vi "fpga_ARC Core (32ch).vi"(0 "data input":i32, 1 "ARC Constants":T3={"bufsize"=512, "bufsize-1"=511, "NChan"=8, "NChan-1"=7, "1/2SymPeriods"=10, "Neg1/2SymPeriods"=-10, "polyOrder-1"=4, "maxDec-1"=24}, 2 "timestamp&count":T1 {"TAI timestamp" format="%.42g"}, 5 "data valid":bool, 7 "resample position [U64.16]":fxp<+,64,16>, 9 "stepsize [U64.8]":fxp<+,64,8>, 11 "position valid":bool, 12 "Ready for output":bool, 13 "Frequency":fxp<+,32,8> format="%.27g") -> (3 "FIFO timeout?":bool, 4 "resample data":T2 {"frequency" format="%.59g"; "Resample position" format="%.53g"; "even-angle signal" format="%.30g"}, 6 "timestamp&count":T1, 8 "muti_ch position valid?":bool, 14 "ready for input":bool, 15 "output valid":bool)   [LabVIEW 2014, in "NI_EP_Resample_FPGA.lvlib"]
uses:
  <vilib>/addons/Electrical Power/PQ/Resampling/NI_EP_Resample_FPGA.lvlib
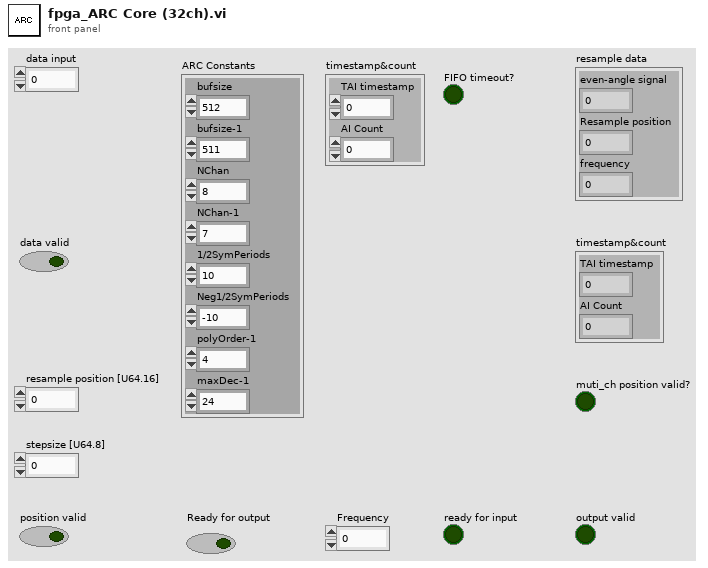
[diagram p1: front panel]
types:
  T1 = cluster{"TAI timestamp":fxp<+,64,32>, "AI Count":u16}
  T2 = cluster{"even-angle signal":fxp<+/-,32,3>, "Resample position":fxp<+,64,16>, "frequency":fxp<+,32,8>}
  T3 = cluster{"bufsize":u16, "bufsize-1":u16, "NChan":u8, "NChan-1":u8, "1/2SymPeriods":i8, "Neg1/2SymPeriods":i8, "polyOrder-1":u8, "maxDec-1":u8}
  T4 = cluster{"sample position":u16, "coef [I32.2]":fxp<+/-,32,2>, "last tap":bool}
  T5 = cluster{"even-angle signal[I32.3]":fxp<+/-,32,3>, "resample position":fxp<+,64,16>, "frequency":fxp<+,32,8>}
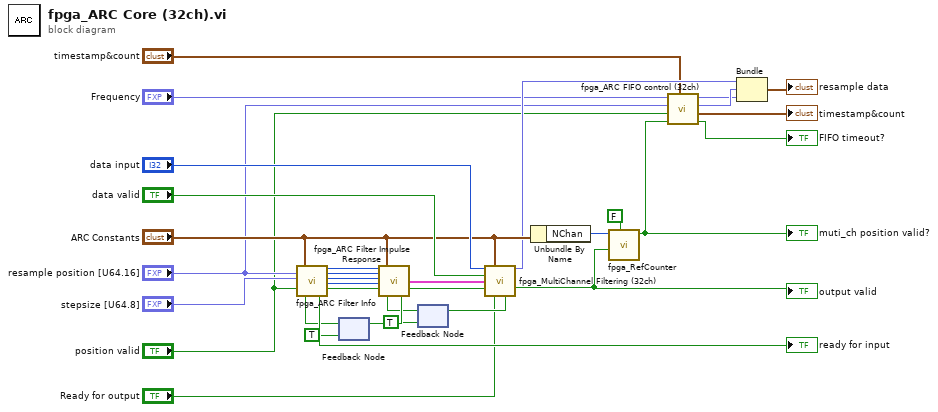
[diagram p0: block diagram]
diagram:
  n1 = feedback #1(TRUE ("ready for input")) -> (w30:bool)
  n2 = call <vilib>:"fpga_ARC Filter Info.vi"("resample position [U64.16]"="resample position [U64.16]", "stepsize [U64.8]"="stepsize [U64.8]", "input valid"="position valid", "ARC Constants"="ARC Constants", "ready for output"=w30) -> ("ready for input"=→"ready for input":bool, "Initial position"=w28:u16, "Initial offset"=w32:u32, "Number of taps"=w26:u16, "filterStepSize[U32.0]"=w31:u32, "output valid"=w27:bool)  [unwired: 1 in, 8 out]
  n3 = feedback #2(TRUE ("ready for filter")) -> (w25:bool)
  n4 = call <vilib>:"fpga_ARC Filter Impulse Response.vi"("Initial position"=w28, "Initial offset"=w32, "Number of taps"=w26, "filterStepSize[U32.0]"=w31, "input valid"=w27, "ARC Constants"="ARC Constants", "ready for output"=w25) -> ("ready for input"=w29:bool, "filter info"=w22:T4, "output valid"=w23:bool)  [unwired: 10 out]
  n5 = feedback-in #1(w29) -> ()
  n6 = call <vilib>:"fpga_MultiChannel Filtering (32ch).vi"("data input"="data input", "ARC Constants"="ARC Constants", "data valid"="data valid", "filter info"=w22, "filter valid"=w23, "Ready for output"="Ready for output") -> ("even-angle signal[I32.3]"=w13:fxp<+/-,32,3>, "output valid"=w10:bool, "ready for filter"=w24:bool)  [unwired: 7 in]
  "output valid" <- w10
  n7 = feedback-in #2(w24) -> ()
  n8 = Unbundle By Name("ARC Constants") -> ("NChan"=w12:u8)
  n9 = call <vilib>:"fpga_RefCounter.vi"("reset"=FALSE, "input valid?"=w10, "NChan"=w12) -> ("Multichannel enable"=w6:bool)  [unwired: 7 in, 1 out]
  "muti_ch position valid?" <- w6
  n10 = call <vilib>:"fpga_ARC FIFO control (32ch).vi"("timestamp&count"="timestamp&count", "Read FIFO"=w6, "write FIFO"="position valid", "resample position"="resample position [U64.16]", "frequency"="Frequency") -> ("FIFO time out?"=→"FIFO timeout?":bool, "timestamp&count"=→"timestamp&count":T1, "resample position"=w5:fxp<+,64,16>, "frequency"=w4:fxp<+,32,8>)  [unwired: 3 in]
  n11 = Bundle("even-angle signal[I32.3]"=w13, "resample position"=w5, "frequency"=w4) -> (→"resample data":T5)  [unwired: 1 in]
